vi "Test PPL Class.vi"(8 "error in (no error)":errorcluster, 10 "Class Path":path, 11 "PPL Class Test Plugin in":refnum<class "PPL Class Test Plugin.lvclass">) -> (0 "error out":errorcluster)   [LabVIEW 2019, in "ProjectBuilder.lvlib" / "PPL Class Test Plugin.lvclass"]
doc: "Override to test a class. Set error on \"error out\" to fail test.\n\nThe default implementation does nothing"
uses:
  PPL Class Test Plugin.lvclass
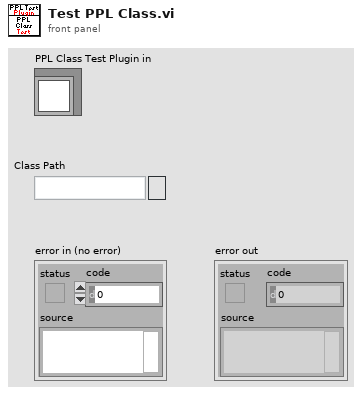
[diagram p1: front panel]
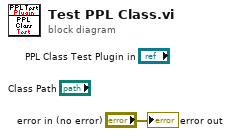
[diagram p0: block diagram]
diagram:
  "error out" <- "error in (no error)"
